vi "5-InitialAllHardware.vi"(8 "error in (no error)":errorcluster, 11 "AllControls IN":T1) -> (3 "InitalResult":bool[](array[boolean]))   [LabVIEW 2017]
uses:
  Ctrls/AllControls.ctl
  Thorlabs.MotionControl.Controls.dll
  Thorlabs.MotionControl.IntegratedStepperMotorsCLI.dll
  <vilib>/Instr/_visa.llb/VISA Configure Serial Port (Instr).vi
panel:
  in  "LongTravelStageControl":refnum<k24>(container)
  in  "SerialNumber":string
  out "error out":errorcluster
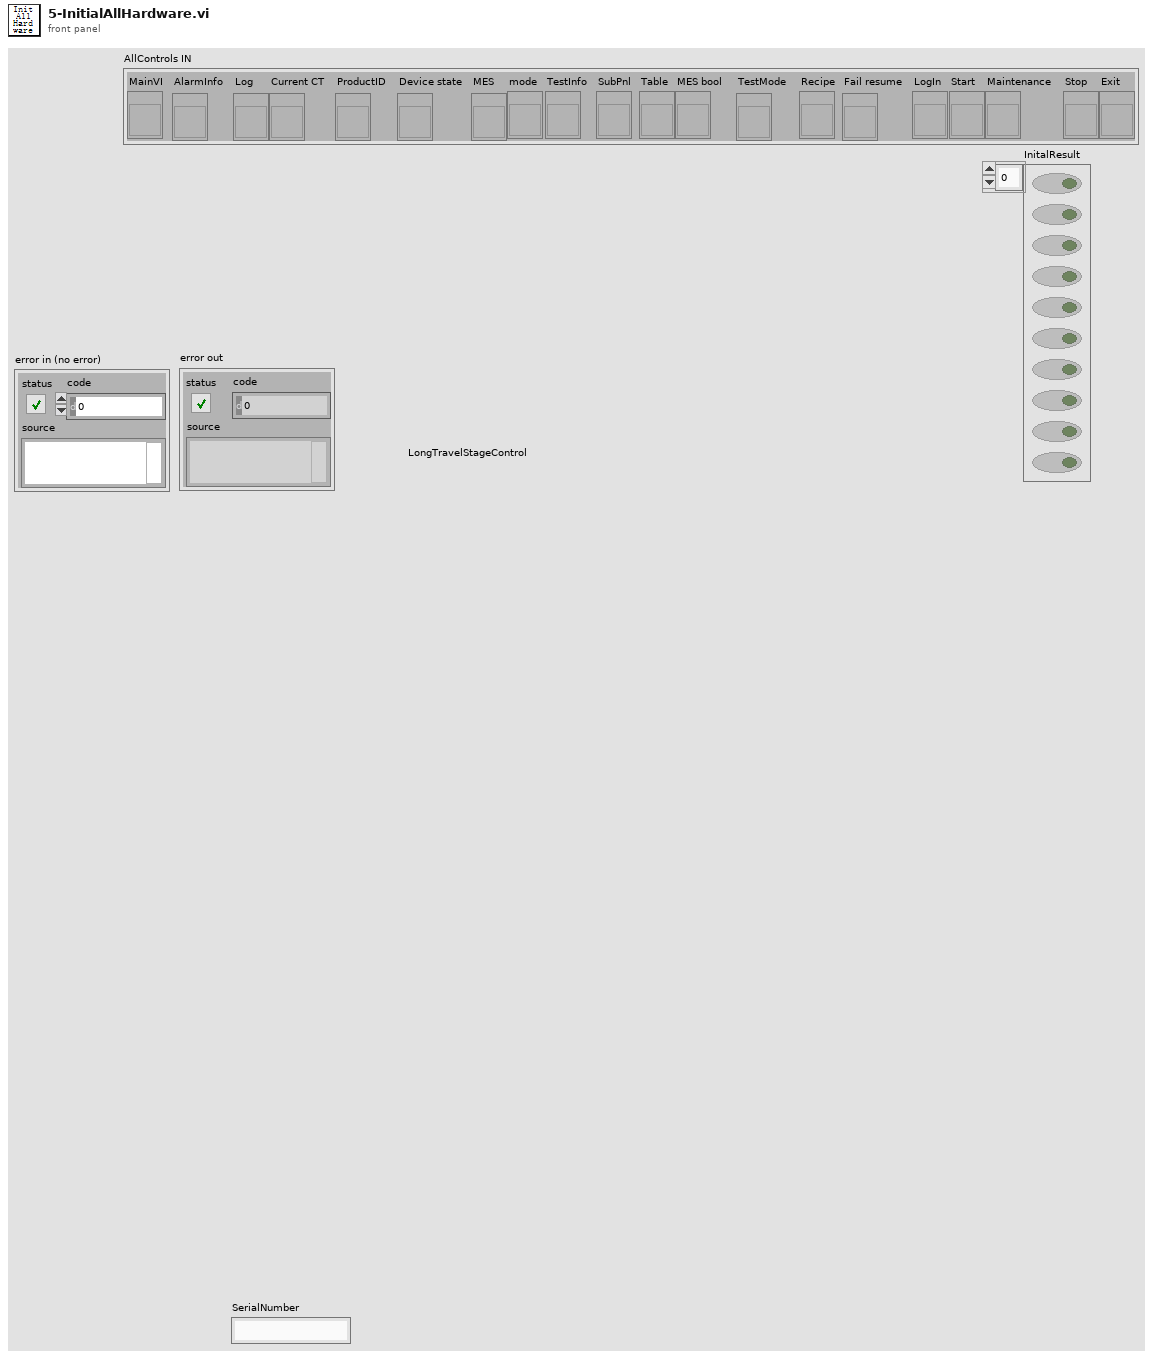
[diagram p1: front panel]
types:
  T1 = typedef "AllControls.ctl" = cluster{"MainVI":refnum<vi>, "AlarmInfo":refnum<vi>, "Log":refnum<vi>, "Current CT":refnum<vi>, "ProductID":refnum<vi>, "Device state":refnum<vi>, "MES":refnum<vi>, "mode":refnum<vi>, "TestInfo":refnum<vi>, "SubPnl":refnum<vi>, "Table":refnum<vi>, "MES bool":refnum<vi>, "TestMode":refnum<vi>, "Recipe":refnum<vi>, "Fail resume":refnum<vi>, "LogIn":refnum<vi>, "Start":refnum<vi>, "Maintenance":refnum<vi>, "Stop":refnum<vi>, "Exit":refnum<vi>}
  T2 = typedef "HD Config.ctl" = cluster{" PC":cluster{"PC Address":u8[], "PC Port":i32}, "FCO":cluster{"COM":refnum<visa-resource-name>, "Baudrate":u32}, "DC Power ":cluster{"COM":refnum<visa-resource-name>, "Baudrate":u32}, "PW3336":cluster{"COM":refnum<visa-resource-name>, "Baudrate":u32}, "Lefoo":cluster{"COM":refnum<visa-resource-name>, "Baudrate":u32}, "Tempt&Hum":cluster{"COM":refnum<visa-resource-name>, "Baudrate":u32}, "DIPC":cluster{"COM":refnum<visa-resource-name>}, "Daemon":cluster{"IP Address":string, "Port":u16, "Retry":u16}, "NFC_Cmd":cluster{"COM":refnum<visa-resource-name>, "Baudrate":u32}, "Fail_resume_mode":bool, "GRR":bool, "NFC _Serial":cluster{"COM":refnum<visa-resource-name>, "Baudrate":u32}}
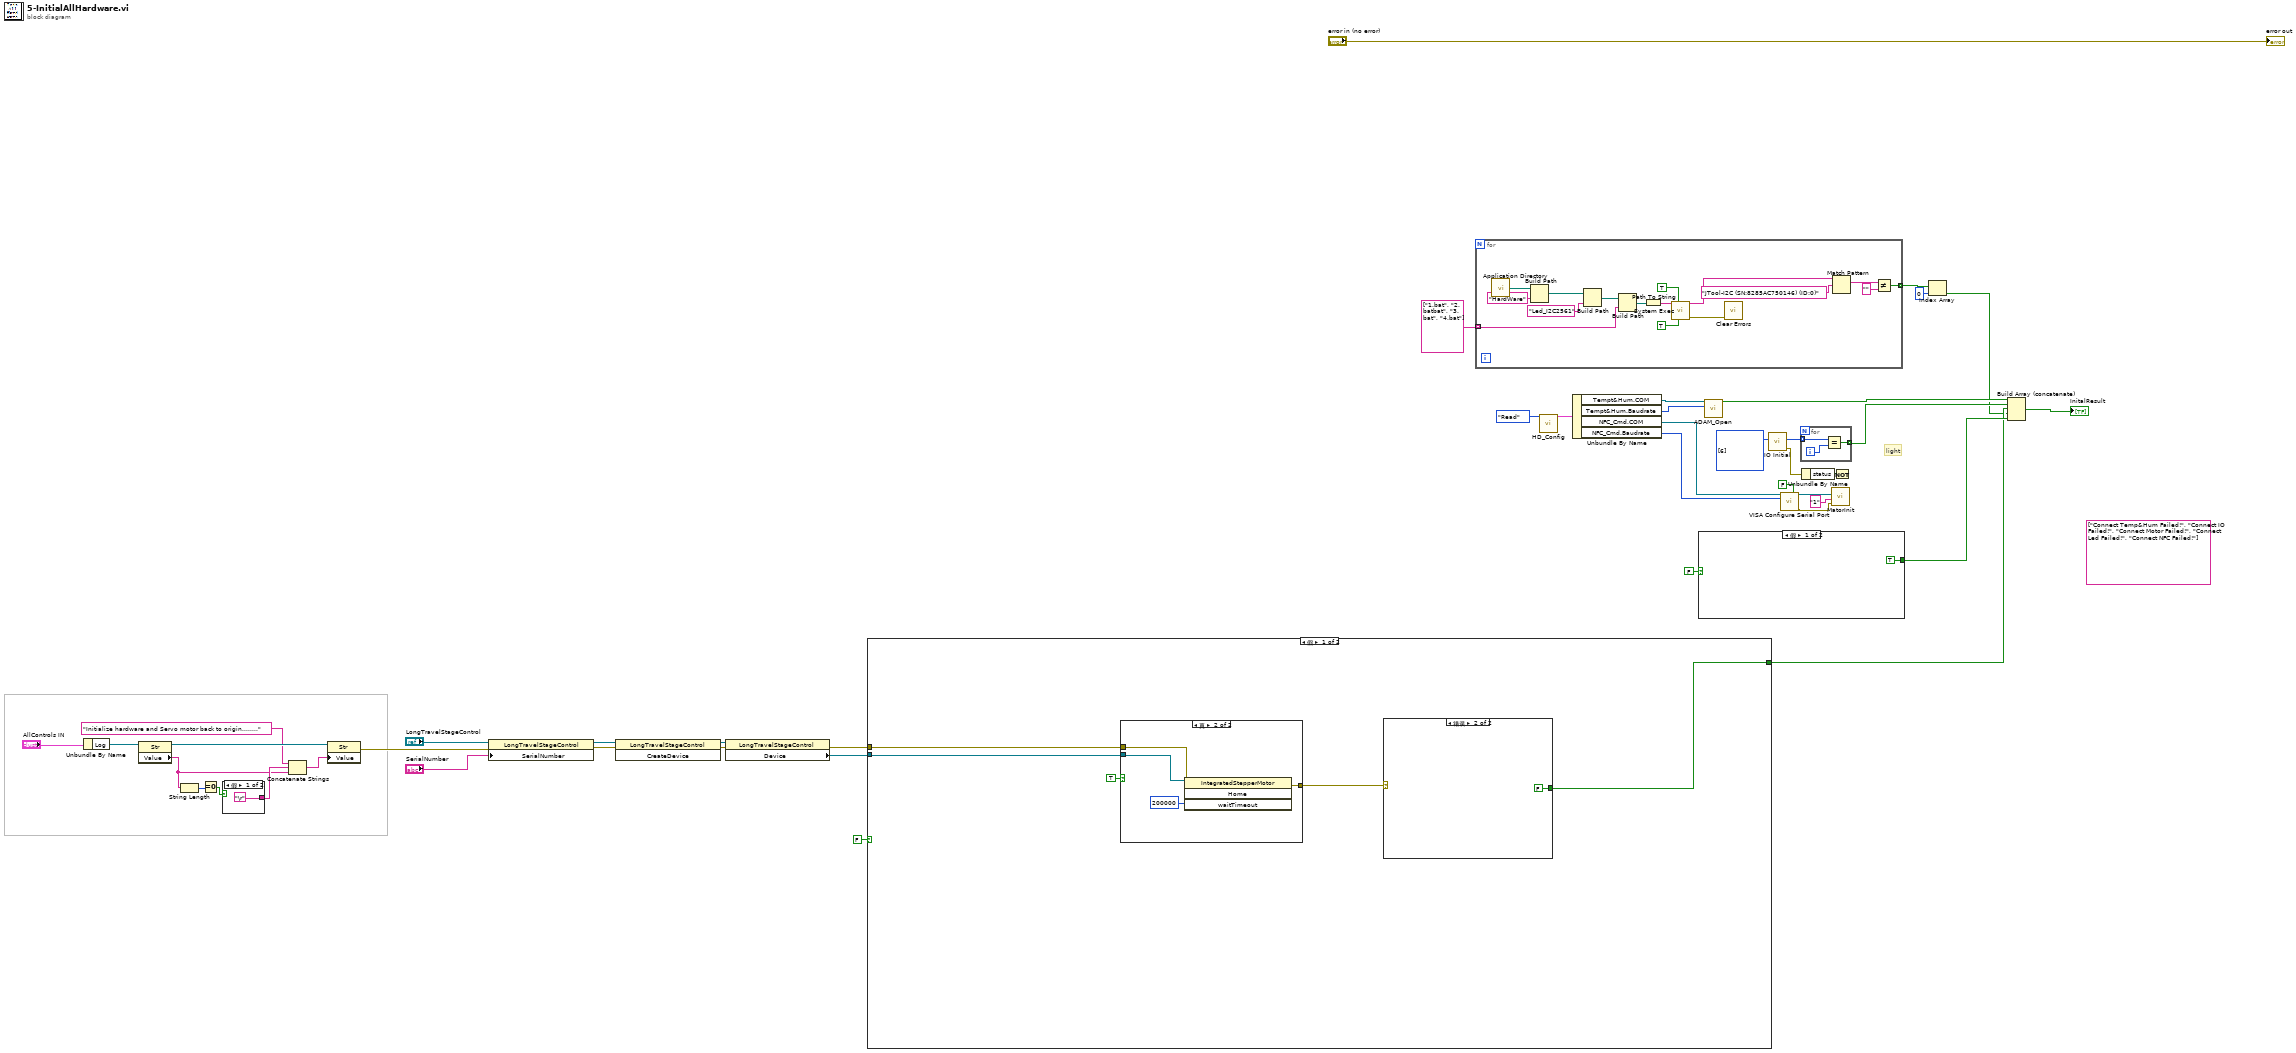
[diagram p0: block diagram]
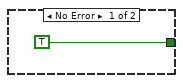
[diagram p3: hidden frame]
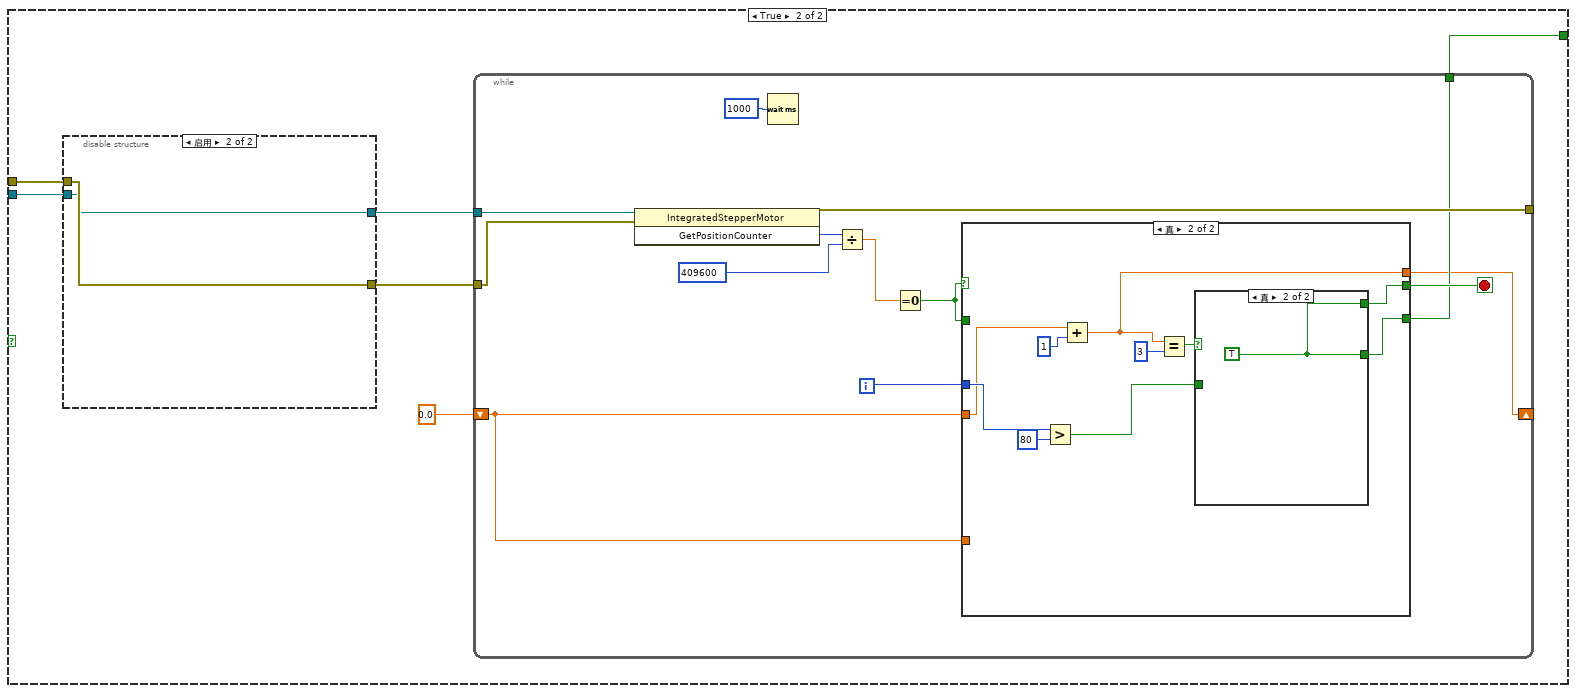
[diagram p4: hidden frame]
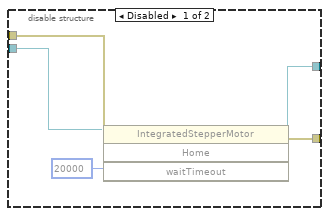
[diagram p5: hidden frame]
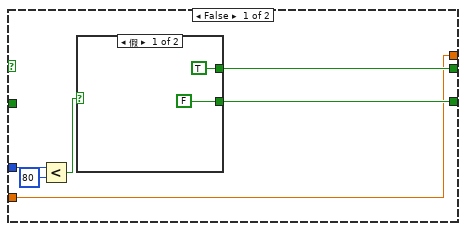
[diagram p6: hidden frame]
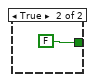
[diagram p7: hidden frame]
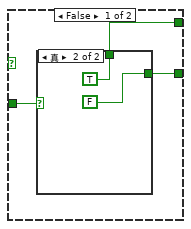
[diagram p8: hidden frame]
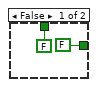
[diagram p9: hidden frame]
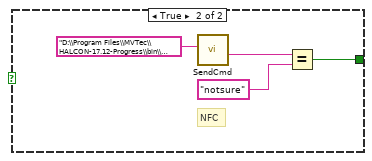
[diagram p10: hidden frame]
diagram:
  (unwired) string[] ["Connect Temp&Hum Failed!", "Connect IO Failed!", "Connect Motor Failed!", "Connect Led Failed!", "Connect NFC Failed!"]
  w40 = u16[] [6] items=["PCI-7230"=6, "PCI-7432"=16, "PCI-7433"=17, "PCI-7434"=18, "PCI-7442"=37] ("CardType")
  # "light"
  n1 = Unbundle By Name("AllControls IN") -> ("Log"=w33:refnum<vi>)
  n2 = property class="Str"(reference=w33) -> (reference out=w35:refnum<vi>, "Value"=w28:string)  [unwired: 1 in, 1 out]
  n3 = String Length(string=w28) -> (length=w30:i32)
  n4 = Equal To 0?(x=w30) -> (x = 0?=w31:bool)
  n5 = case shown="假" w31 {
    tunnel: ["\r" _] -> w29
    frame False {
    }
    frame True {
    }
  }
  n6 = Concatenate Strings("Initialize hardware and Servo motor back to origin........" ("字符串"), w29, w28) -> (w32:string)
  n7 = property class="Str"(reference=w35, "Value"=w32) -> (error out=w16:errorcluster)  [unwired: 1 in, 1 out]
  n8 = property class="LongTravelStageControl"(reference="LongTravelStageControl", error in=w16, "SerialNumber"="SerialNumber") -> (reference out=w6:refnum<k24>, error out=w4:errorcluster)
  n9 = invoke class="LongTravelStageControl" method="CreateDevice"(reference=w6, error in=w4) -> (reference out=w5:refnum<k24>, error out=w3:errorcluster)  [unwired: 1 in, 1 out]
  n10 = property class="LongTravelStageControl"(reference=w5, error in=w3) -> (error out=w14:errorcluster, "Device"=w13:refnum<k24>)  [unwired: 1 out]
  n11 = case shown="假" FALSE {
    tunnel: [w48 w63] -> w15
    tunnel: w14 -> [w49 w62]
    tunnel: w13 -> [w50 w61]
    frame False {
      n12 = case shown="真" TRUE {
        tunnel: w50 -> [_ w55]
        tunnel: w49 -> [w51 w54]
        tunnel: [w51 w52] -> w47
        frame False {
        }
        frame True {
          n13 = invoke class="IntegratedStepperMotor" method="Home"(reference=w55, error in=w54, "waitTimeout"=200000) -> (error out=w52:errorcluster)  [unwired: 1 in, 3 out]
        }
      }
      n14 = case shown="错误" w47 {
        tunnel: [TRUE FALSE] -> w48
        frame No Error {
        }
        frame Error {
        }
      }
    }
    frame True {
      n15 = disable-structure shown="启用" {
        disable-tunnel: w62 -> [w67 w70]
        disable-tunnel: w61 -> [w66 w69]
        disable-tunnel: [w65 w69] -> w60
        disable-tunnel: [w64 w70] -> w59
        frame Disabled {
          n16 = invoke class="IntegratedStepperMotor" method="Home"(reference=w66, error in=w67, "waitTimeout"=20000) -> (reference out=w65:refnum<k24>, error out=w64:errorcluster)  [unwired: 1 in, 2 out]
        }
        frame Enabled {
        }
      }
      n17 = while {
        tunnel: [w81] -> _
        tunnel: [w73] -> w63
        tunnel: w60 -> [w78]
        tunnel: w59 -> [w77]
        shift-right: [w71] -> _
        shift-left: 0.0 -> [w72]
        i -> [w74]
        stop <- w75 stop-if-true
        n18 = invoke class="IntegratedStepperMotor" method="GetPositionCounter"(reference=w78, error in=w77) -> (error out=w81:errorcluster, "GetPositionCounter"=w80:i32)  [unwired: 1 in, 1 out]
        n19 = Wait (ms)(milliseconds to wait=u32 1000) -> ()  [unwired: 1 out]
        n20 = Divide(x=w80, y=409600 ("GetPositionCounter")) -> (x/y=w79:dbl)
        n21 = Equal To 0?(x=w79) -> (x = 0?=w76:bool)
        n22 = case shown="真" w76 {
          tunnel: w76 -> [_ _]
          tunnel: [w89 w96] -> w75
          tunnel: w74 -> [w88 w101]
          tunnel: [w85 w98] -> w73
          tunnel: w72 -> [_ _]
          tunnel: w72 -> [w84 w95]
          tunnel: [w84 w93] -> w71
          frame False {
            n23 = Less?(x=w88, y=80) -> (x < y?=w86:bool)
            n24 = case shown="假" w86 {
              tunnel: [TRUE FALSE] -> w89
              tunnel: [FALSE _] -> w85
              frame False {
              }
              frame True {
              }
            }
          }
          frame True {
            n25 = Greater?(x=w101, y=80) -> (0:w97:bool)
            n26 = Add(x=w95, y=1) -> (x+y=w93:dbl)
            n27 = Equal?(x=w93, y=u32 3) -> (x = y?=w99:bool)
            n28 = case shown="真" w99 {
              tunnel: [w103 w110] -> w98
              tunnel: w97 -> [w105 _]
              tunnel: [w104 w110] -> w96
              frame False {
                n29 = case shown="真" w105 {
                  tunnel: [FALSE TRUE] -> w104
                  tunnel: [FALSE FALSE] -> w103
                  frame False {
                  }
                  frame True {
                  }
                }
              }
              frame True {
                w110 = TRUE
              }
            }
          }
        }
      }
    }
  }
  n30 = for {
    tunnel: string[] ["1.bat", "2.batbat", "3.bat", "4.bat"] -> [w115] mode=indexing
    tunnel: [w111] -> w9 mode=indexing
    n31 = call <vilib>:"Application Directory.vi"() -> ("Application Directory"=w120:path)
    n32 = Build Path(base path=w120, name or relative path="HardWare") -> (appended path=w118:path)
    n33 = Build Path(base path=w118, name or relative path="Led_I2C2561") -> (appended path=w116:path)
    n34 = Build Path(base path=w116, name or relative path=w115) -> (appended path=w114:path)
    n35 = Path To String(path=w114) -> (string=w113:string)
    n36 = call <vilib>:"System Exec.vi"("run minimized? (F)"=TRUE, "wait until completion? (T)"=TRUE, "command line"=w113) -> ("error out"=w112:errorcluster, "standard output"=w124:string)  [unwired: 3 in, 4 out]
    n37 = call <vilib>:"Clear Errors.vi"("error in (no error)"=w112) -> ()  [unwired: 5 in, 2 out]
    n38 = Match Pattern(string=w124, regular expression="JTool-I2C (SN:8285AC750146) (ID:0)") -> (match substring=w122:string)  [unwired: 1 in, 3 out]
    n39 = Not Equal?(x=w122, y="") -> (x != y?=w111:bool)
  }
  n40 = call "HD_Config.vi"("Step"=enum16{"Initial", "Write", "Read"}."Read") -> ("HD Config out"=w41:T2)  [unwired: 9 in, 1 out]
  n41 = Unbundle By Name(w41) -> ("Tempt&Hum.COM"=w26:refnum<visa-resource-name>, "Tempt&Hum.Baudrate"=w25:u32, "NFC_Cmd.COM"=w21:refnum<visa-resource-name>, "NFC_Cmd.Baudrate"=w11:u32)
  n42 = case shown="假" FALSE {
    tunnel: [TRUE w128] -> w18
    frame False {
    }
    frame True {
      # "NFC"
      n43 = call "SendCmd.vi"("exe"="D:\\Program Files\\MVTec\\HALCON-17.12-Progress\\bin\\x64-win64\\hdevelop.exe") -> ("standard output"=w130:string)  [unwired: 7 in, 3 out]
      n44 = Equal?(x=w130, y="notsure") -> (x = y?=w128:bool)
    }
  }
  n45 = call "ADAM_Open.vi"("port"=w25, "VISA resource name"=w26) -> ("status"=w24:bool)  [unwired: 8 in, 1 out]
  n46 = call "IO Initial.vi"("CardType"=w40) -> ("error out"=w37:errorcluster, "IO f"=w39:i16[])  [unwired: 9 in]
  n47 = call-poly "VISA Configure Serial Port"("VISA resource name"=w21, "Enable Termination\nChar (T)"=FALSE ("Enable Termination\nChar (T)"), "baud rate (9600)"=w11) -> ("VISA resource name out"=w20:refnum<visa-resource-name>, "error out"=w19:errorcluster)  [unwired: 6 in, 5 out]
  n48 = for {
    tunnel: w39 -> [w134] mode=indexing
    tunnel: [w132] -> w38 mode=indexing
    i -> [w133]
    n49 = Equal?(x=w134, y=w133) -> (x = y?=w132:bool)
  }
  n50 = Unbundle By Name(w37) -> ("status"=w36:bool)
  n51 = call "MatorInit.vi"("错误输入（无错误）"=w19, "Chan Ident"="1", "VISA资源名称"=w20) -> ()  [unwired: 8 in, 1 out]
  n52 = Not(x=w36) -> ()  [unwired: 1 out]
  n53 = Index Array(array=w9, index=0) -> (element=w7:bool)
  n54 = Build Array (concatenate)(w24, w38, w15, w7, w18) -> (→"InitalResult":bool[])
  "error out" <- "error in (no error)"
